vi "Begin.vi"(11 "Image Size":T1=enum."160x120") -> (0 "error out":errorcluster)   [LabVIEW 2012]
doc: "Called before other user functions, this VI is expected to open initial I/O refnums, load in file data, and do all program initialization. Notice that the <B>error out</B> terminal is simply used for data flow. Wiring it to other structures or subVIs ensures that this VI runs first."
uses:
  <vilib>/Rock Robotics/WPI/Camera/WPI_CameraImageSize.ctl
  <vilib>/Rock Robotics/SystemInterfaces/Utilities/FPGA_UtilitiesLED State.ctl
  <vilib>/Rock Robotics/WPI/Joystick/WPI_JoystickDeviceEnum.ctl
  <vilib>/Rock Robotics/SystemInterfaces/DIO/FPGA_DIOChannel.ctl
  <vilib>/Rock Robotics/SystemInterfaces/AI/FPGA_AIChannel.ctl
  <vilib>/Rock Robotics/WPI/Encoder/WPI_EncoderDevRef.ctl
  <vilib>/Rock Robotics/SystemInterfaces/Encoder/FPGA_EncoderIdx.ctl
  <vilib>/Rock Robotics/SystemInterfaces/Counter/FPGA_CounterCtrSystemIndex.ctl
  <vilib>/Rock Robotics/WPI/Encoder/WPI_EncoderType.ctl
  <vilib>/Rock Robotics/WPI/AnalogChannel/WPI_AnalogChannelDevRef.ctl
  <vilib>/Rock Robotics/SystemInterfaces/Typedef/FPGA_TypedefAnalogModule.ctl
  <vilib>/Rock Robotics/WPI/MotorControl/WPI_MotorControlDeviceRef.ctl
  <vilib>/Rock Robotics/SystemInterfaces/Typedef/FPGA_TypedefDigitalModule.ctl
  <vilib>/Rock Robotics/SystemInterfaces/DIO/FPGA_DIOPWMChannel.ctl
  <vilib>/Rock Robotics/WPI/PWM/WPI_PWMDeadband.ctl
  <vilib>/Rock Robotics/WPI/CAN/Jaguar/SubVIs/WPI_CANJaguar_ControlMode.ctl
  <vilib>/Rock Robotics/WPI/PWM/WPI_PWMTransform_ConPane.ctl
  <vilib>/Rock Robotics/SystemInterfaces/Utilities/FPGA_UtilitiesLED Source.ctl
  <vilib>/Utility/file.llb/Read From Spreadsheet File (DBL).vi
  Globals/Pot Home Values.vi
  Globals/Robot Jaguars.vi
  Globals/Encoders Global.vi
  Globals/Potentiometers.vi
  Globals/Are We Calibrating Steering.vi
  Globals/Are We Calibrating Actuator.vi
  Globals/Jaguar Commands.vi
  Globals/Autonomous Joystick Emulation.vi
  Globals/Autonomous Tipping.vi
  Globals/Actuator Home Position.vi
  Globals/Max Tipper Angle.vi
  <vilib>/Rock Robotics/WPI/Camera/WPI_CameraWhite Balance Values.ctl
  <vilib>/Rock Robotics/WPI/Camera/WPI_CameraExposure Values.ctl
  <vilib>/Rock Robotics/WPI/Camera/WPI_CameraFrameRate.ctl
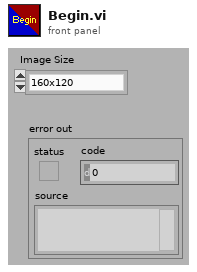
[diagram p1: front panel]
types:
  T1 = typedef "WPI_CameraImageSize.ctl" = enum16{"640x480", "320x240", "160x120"}
  T2 = typedef "FPGA_DIOChannel.ctl" = enum8{"DIO 1", "DIO 2", "DIO 3", "DIO 4", "DIO 5", "DIO 6", "DIO 7", "DIO 8", "DIO 9", "DIO 10", "DIO 11", "DIO 12", "DIO 13", "DIO 14", "Invalid"}
  T3 = typedef "FPGA_TypedefDigitalModule.ctl" = enum16{"Digital Module 1", "Digital Module 2"}
  T4 = typedef "FPGA_AIChannel.ctl" = enum8{"AI 1", "AI 2", "AI 3", "AI 4", "AI 5", "AI 6", "AI 7", "AI 8", "Invalid"}
  T5 = typedef "WPI_EncoderType.ctl" = enum16{"1x", "2x", "4x"}
  T6 = typedef "WPI_MotorControlDeviceRef.ctl" = cluster{"DeviceStatus":errorcluster, "Type":enum16{"PWM", "CAN"}, "PWM":cluster{"Digital Module":T3, "PWM Channel":T7, "DeadBand":T8}, "CAN":cluster{"Device Number":u8, "Control Mode":T9, "Semaphore":T10, "Max Vout":dbl}, "Invert":bool, "TransformRef":T11, "InvTransformRef":T11}
  T7 = typedef "FPGA_DIOPWMChannel.ctl" = enum8{"PWM 1", "PWM 2", "PWM 3", "PWM 4", "PWM 5", "PWM 6", "PWM 7", "PWM 8", "PWM 9", "PWM 10", "Invalid"}
  T8 = typedef "WPI_PWMDeadband.ctl" = cluster{"Name":string, "maxPositivePwm":i32, "minPositivePwm":i32, "centerPwm":i32, "maxNegativePwm":i32, "minNegativePwm":i32, "angularRange":u16}
  T9 = typedef "WPI_CANJaguar_ControlMode.ctl" = enum8{"Percent VBus", "Current", "Speed", "Position", "Voltage"}
  T10 = typedef "Semaphore RefNum" = refnum<k1>
  T11 = typedef "WPI_PWMTransform_ConPane.ctl" = refnum<vi>
  T12 = cluster{"MotorControlDevRef":T6, "MotorControlDevRef":T6, "MotorControlDevRef":T6, "MotorControlDevRef":T6, "MotorControlDevRef":T6, "MotorControlDevRef":T6, "MotorControlDevRef":T6, "MotorControlDevRef":T6}
  T13 = typedef "WPI_AnalogChannelDevRef.ctl" = cluster{"DevStatus":errorcluster, "Analog Module":T14, "Analog Channel":T4}
  T14 = typedef "FPGA_TypedefAnalogModule.ctl" = enum16{"Analog Module 1", "Analog Module 2"}
  T15 = cluster{"Front Left":T13, "Front Right":T13, "Rear Left":T13, "Rear Right":T13, "Actuator":T13}
  T16 = typedef "WPI_EncoderDevRef.ctl" = cluster{"DevStatus":errorcluster, "EncoderIndex":T17, "CounterIndex":T18, "DistancePerCount":dbl, "Decoding Type":T5}
  T17 = typedef "FPGA_EncoderIdx.ctl" = enum8{"Enc 0", "Enc 1", "Enc 2", "Enc 3", "Invalid"}
  T18 = typedef "FPGA_CounterCtrSystemIndex.ctl" = enum8{"Ctr 0", "Ctr 1", "Ctr 2", "Ctr 3", "Ctr 4", "Ctr 5", "Ctr 6", "Ctr 7", "Invalid"}
  T19 = cluster{"Front Left":T16, "Front Right":T16, "Rear Left":T16, "Rear Right":T16, "Shooter":T16}
  T20 = typedef "WPI_JoystickDeviceEnum.ctl" = enum16{"USB 1", "USB 2", "USB 3", "USB 4", "Kinect 1", "Kinect 2"}
  T21 = typedef "FPGA_UtilitiesLED State.ctl" = enum16{"Off", "On", "Toggle"}
  T22 = typedef "FPGA_UtilitiesLED Source.ctl" = enum16{"User LED", "FPGA LED"}
  T23 = typedef "WPI_JoystickDevRef.ctl" = cluster{"Device":T20}
  T24 = typedef "WPI_CameraFrameRate.ctl" = u32
  T25 = typedef "WPI_CameraExposure Values.ctl" = enum16{"Auto", "Flicker-free 50 Hz", "Flicker-free 60 Hz", "Hold current"}
  T26 = typedef "WPI_CameraWhite Balance Values.ctl" = enum16{"Auto", "Fixed indoor", "Fixed outdoor 1", "Fixed outdoor 2", "Fixed fluorescent 1", "Fixed fluorescent 2", "Hold current"}
  T27 = typedef "WPI_CameraDevRef.ctl" = cluster{"Camera Address":string, "CameraStatus":errorcluster, "Acquire Image Notifier":refnum<notifier>}
  T28 = typedef "WPI_DigitalInputDevRef.ctl" = cluster{"DevStatus":errorcluster, "DIO Channel":T2, "Digital Module":T3}
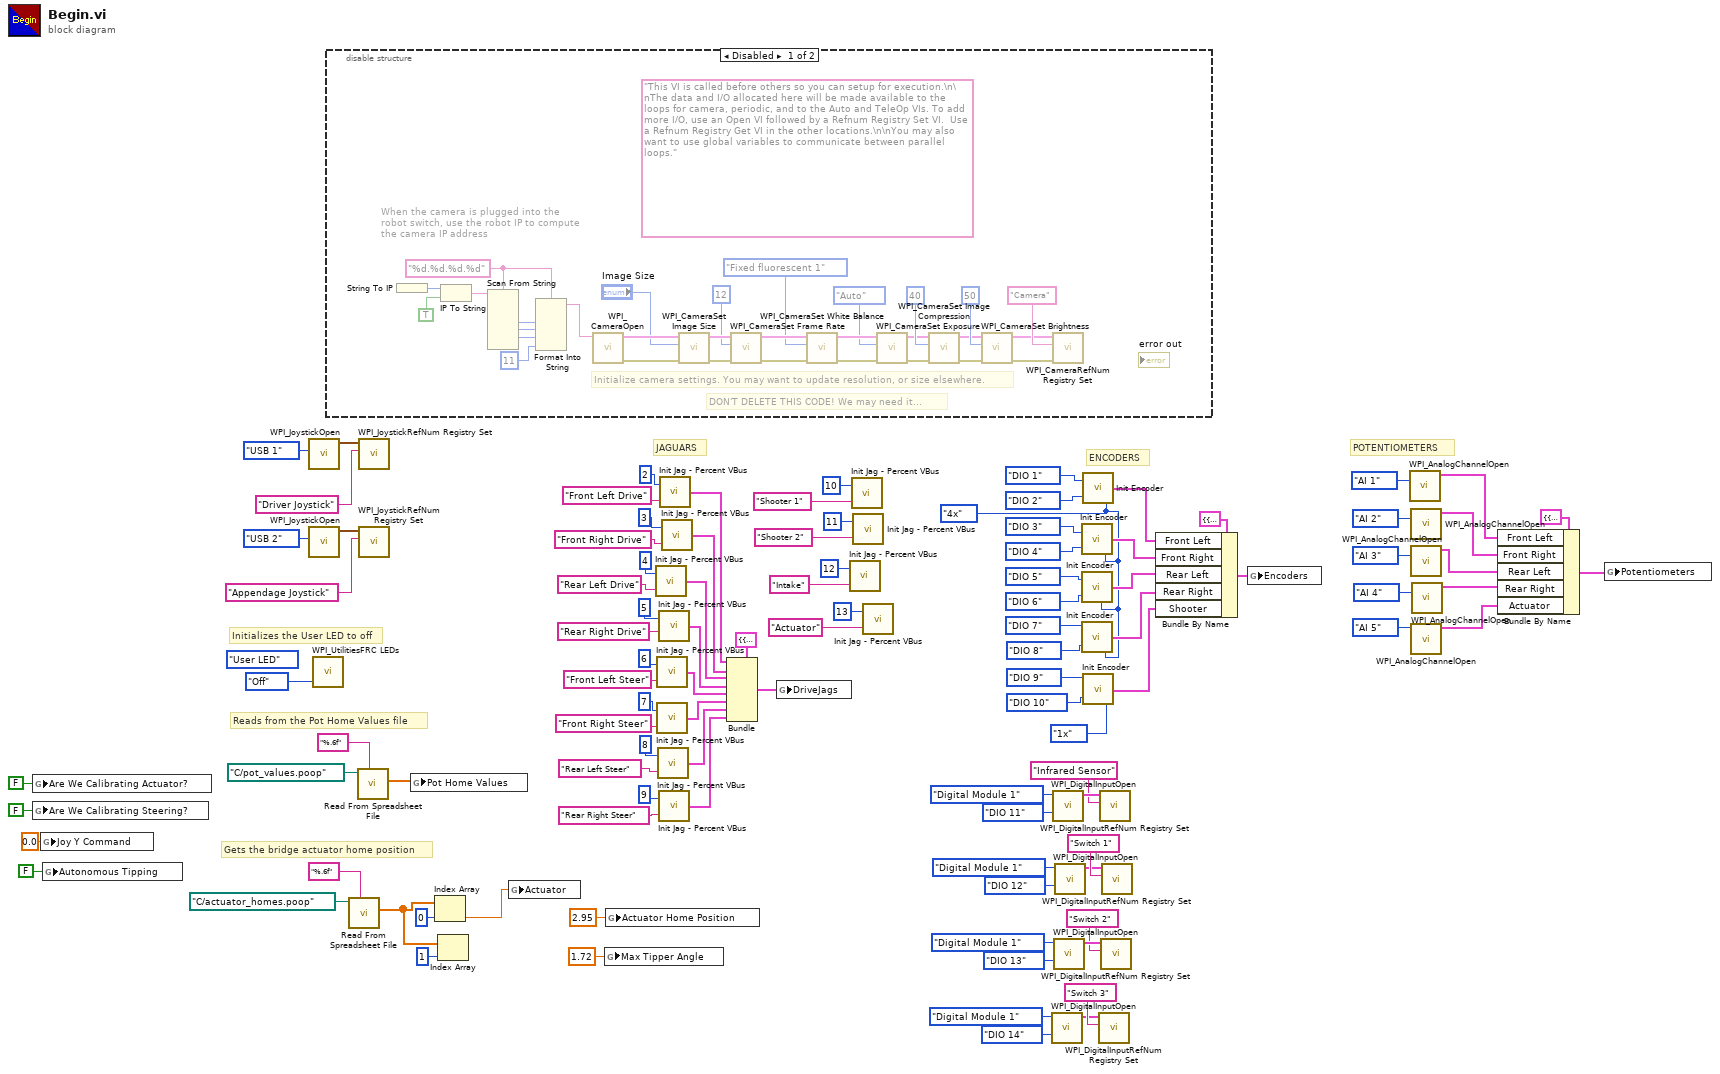
[diagram p0: block diagram]
diagram:
  w64 = WPI_EncoderType."4x" ("Decoding Type")
  (unwired) FPGA_UtilitiesLED_Source."User LED" ("LED Type")
  # "Gets the bridge actuator home position"
  # "JAGUARS"
  # "POTENTIOMETERS"
  # "ENCODERS"
  # "Reads from the Pot Home Values file"
  # "Initializes the User LED to off"
  n1 = global write "Are We Calibrating Actuator.vi" "Are We Calibrating Actuator?"(FALSE ("Are We Calibrating Actuator?")) -> ()
  n2 = global write "Are We Calibrating Steering.vi" "Are We Calibrating Steering?"(FALSE ("Are We Calibrating Steering?")) -> ()
  n3 = global write "Autonomous Joystick Emulation.vi" "Joy Y Command"(0.0 ("Joy Y Command")) -> ()
  n4 = global write "Autonomous Tipping.vi" "Autonomous Tipping"(FALSE ("Autonomous Tipping")) -> ()
  n5 = call <vilib>:"WPI_JoystickOpen.vi"("JoystickDevice"=WPI_JoystickDeviceEnum."USB 1") -> ("JoystickDevRef"=w98:T23)  [unwired: 10 in]
  n6 = call <vilib>:"WPI_JoystickOpen.vi"("JoystickDevice"=WPI_JoystickDeviceEnum."USB 2") -> ("JoystickDevRef"=w95:T23)  [unwired: 10 in]
  n7 = call <vilib>:"WPI_UtilitiesFRC LEDs.vi"("State"=FPGA_UtilitiesLED_State."Off") -> ()  [unwired: 9 in, 2 out]
  n8 = disable-structure shown="Disabled" {
    frame Disabled {
      w105 = "%d.%d.%d.%d" ("format string")
      (unwired) "This VI is called before others so you can setup for execution.\n\nThe data and I/O allocated here will be made available to the loops for camera, periodic, and to the Auto and TeleOp VIs. To add more I/O, use an Open VI followed by a Refnum Registry Set VI.  Use a Refnum Registry Get VI in the other locations.\n\nYou may also want to use global variables to communicate between parallel loops."
      # "DON'T DELETE THIS CODE! We may need it..."
      # "When the camera is plugged into the\nrobot switch, use the robot IP to compute\nthe camera IP address"
      # "Initialize camera settings. You may want to update resolution, or size elsewhere."
      n9 = String To IP() -> (0:w112:u32)  [unwired: 1 in]
      n10 = IP To String(1:TRUE ("dot notation? (F)"), 2:w112) -> (0:w110:string)
      n11 = Scan From String(format string=w105, input string=w110) -> (output 1=w109:i32, output 2=w108:i32, output 3=w107:i32)  [unwired: 7 in, 3 out]
      n12 = Format Into String(format string=w105, w109, w108, w107, 11 ("Compression")) -> (resulting string=w104:string)  [unwired: 2 in, 1 out]
      n13 = call <vilib>:"WPI_CameraOpen.vi"("Camera Address"=w104) -> ("error out"=w124:errorcluster, "CameraDevRef"=w125:T27)  [unwired: 1 in, 8 out]
      n14 = call <vilib>:"WPI_CameraSet Image Size.vi"("error in (no error)"=w124, "Image Size"="Image Size", "CameraDevRef"=w125) -> ("error out"=w123:errorcluster, "CameraDevRef Out"=w126:T27)  [unwired: 7 out]
      n15 = call <vilib>:"WPI_CameraSet Frame Rate.vi"("error in (no error)"=w123, "Frame Rate (fps)"=T24 12, "CameraDevRef"=w126) -> ("error out"=w122:errorcluster, "CameraDevRef Out"=w128:T27)  [unwired: 7 out]
      n16 = call <vilib>:"WPI_CameraSet White Balance.vi"("error in (no error)"=w122, "White Balance"=WPI_CameraWhite_Balance_Values."Fixed fluorescent 1", "CameraDevRef"=w128) -> ("error out"=w121:errorcluster, "CameraDevRef Out"=w127:T27)  [unwired: 7 out]
      n17 = call <vilib>:"WPI_CameraSet Exposure.vi"("error in (no error)"=w121, "Exposure"=WPI_CameraExposure_Values."Auto", "CameraDevRef"=w127) -> ("error out"=w120:errorcluster, "CameraDevRef Out"=w130:T27)  [unwired: 7 out]
      n18 = call <vilib>:"WPI_CameraSet Image Compression.vi"("error in (no error)"=w120, "Compression"=40, "CameraDevRef"=w130) -> ("error out"=w119:errorcluster, "CameraDevRef Out"=w129:T27)  [unwired: 7 out]
      n19 = call <vilib>:"WPI_CameraSet Brightness.vi"("error in (no error)"=w119, "Brightness"=50, "CameraDevRef"=w129) -> ("error out"=w117:errorcluster, "CameraDevRef Out"=w118:T27)  [unwired: 7 out]
      n20 = call <vilib>:"WPI_CameraRefNum Registry Set.vi"("error in (no error)"=w117, "refnum name"="Camera", "CameraDevRef"=w118) -> ()  [unwired: 9 out]
    }
    frame Enabled {
    }
  }
  n21 = call-poly <vilib>:"Read From Spreadsheet File.vi"("format (%.3f)"="%.6f", "file path (dialog if empty)"=path "C:/actuator_homes.poop") -> ("first row"=w35:dbl[])  [unwired: 5 in, 4 out]
  n22 = call-poly <vilib>:"Read From Spreadsheet File.vi"("format (%.3f)"="%.6f", "file path (dialog if empty)"=path "C:/pot_values.poop") -> ("first row"=w100:dbl[])  [unwired: 5 in, 4 out]
  n23 = call <vilib>:"WPI_JoystickRefNum Registry Set.vi"("refnum name"="Driver Joystick", "JoystickDevRef"=w98) -> ()  [unwired: 8 in, 2 out]
  n24 = call <vilib>:"WPI_JoystickRefNum Registry Set.vi"("refnum name"="Appendage Joystick", "JoystickDevRef"=w95) -> ()  [unwired: 8 in, 2 out]
  n25 = global write "Pot Home Values.vi" "Pot Home Values"(w100) -> ()
  n26 = Index Array(array=w35, index=0) -> (element=w33:dbl)
  n27 = Index Array(array=w35, index=1) -> ()  [unwired: 1 out]
  n28 = global write "Jaguar Commands.vi" "Actuator"(w33) -> ()
  n29 = global write "Max Tipper Angle.vi" "Max Tipper Angle"(1.72 ("Max Tipper Angle")) -> ()
  n30 = global write "Actuator Home Position.vi" "Actuator Home Position"(2.95 ("Actuator Home Position")) -> ()
  n31 = call "Init Jag - Percent VBus.vi"("Jag Refnum Name"="Rear Left Drive", "Device Number"=u8 4) -> ("MotorControlDevRef"=w54:T6)
  n32 = call "Init Jag - Percent VBus.vi"("Jag Refnum Name"="Front Left Steer", "Device Number"=u8 6) -> ("MotorControlDevRef"=w3:T6)
  n33 = call "Init Jag - Percent VBus.vi"("Jag Refnum Name"="Front Right Steer", "Device Number"=u8 7) -> ("MotorControlDevRef"=w4:T6)
  n34 = call "Init Jag - Percent VBus.vi"("Jag Refnum Name"="Rear Left Steer", "Device Number"=u8 8) -> ("MotorControlDevRef"=w6:T6)
  n35 = call "Init Jag - Percent VBus.vi"("Jag Refnum Name"="Rear Right Drive", "Device Number"=u8 5) -> ("MotorControlDevRef"=w51:T6)
  n36 = call "Init Jag - Percent VBus.vi"("Jag Refnum Name"="Rear Right Steer", "Device Number"=u8 9) -> ("MotorControlDevRef"=w5:T6)
  n37 = call "Init Jag - Percent VBus.vi"("Jag Refnum Name"="Front Left Drive", "Device Number"=u8 2) -> ("MotorControlDevRef"=w62:T6)
  n38 = call "Init Jag - Percent VBus.vi"("Jag Refnum Name"="Front Right Drive", "Device Number"=u8 3) -> ("MotorControlDevRef"=w57:T6)
  n39 = Bundle(cluster=T12 {"MotorControlDevRef"={"DeviceStatus"={"status"=FALSE, "code"=0, "source"=""}, "Type"=enum."PWM", "PWM"={"Digital Module"=enum."Digital Module 1", "PWM Channel"=enum."PWM 1", "DeadBand"={"Name"="", "maxPositivePwm"=0, "minPositivePwm"=0, "centerPwm"=0, "maxNegativePwm"=0, "minNegativePwm"=0, "angularRange"=0}}, "CAN"={"Device Number"=0, "Control Mode"=enum."Percent VBus", "Semaphore"=refnum, "Max Vout"=0.0}, "Invert"=FALSE, "TransformRef"=refnum, "InvTransformRef"=refnum}, "MotorControlDevRef"={"DeviceStatus"={"status"=FALSE, "code"=0, "source"=""}, "Type"=enum."PWM", "PWM"={"Digital Module"=enum."Digital Module 1", "PWM Channel"=enum."PWM 1", "DeadBand"={"Name"="", "maxPositivePwm"=0, "minPositivePwm"=0, "centerPwm"=0, "maxNegativePwm"=0, "minNegativePwm"=0, "angularRange"=0}}, "CAN"={"Device Number"=0, "Control Mode"=enum."Percent VBus", "Semaphore"=refnum, "Max Vout"=0.0}, "Invert"=FALSE, "TransformRef"=refnum, "InvTransformRef"=refnum}, "MotorControlDevRef"={"DeviceStatus"={"status"=FALSE, "code"=0, "source"=""}, "Type"=enum."PWM", "PWM"={"Digital Module"=enum."Digital Module 1", "PWM Channel"=enum."PWM 1", "DeadBand"={"Name"="", "maxPositivePwm"=0, "minPositivePwm"=0, "centerPwm"=0, "maxNegativePwm"=0, "minNegativePwm"=0, "angularRange"=0}}, "CAN"={"Device Number"=0, "Control Mode"=enum."Percent VBus", "Semaphore"=refnum, "Max Vout"=0.0}, "Invert"=FALSE, "TransformRef"=refnum, "InvTransformRef"=refnum}, "MotorControlDevRef"={"DeviceStatus"={"status"=FALSE, "code"=0, "source"=""}, "Type"=enum."PWM", "PWM"={"Digital Module"=enum."Digital Module 1", "PWM Channel"=enum."PWM 1", "DeadBand"={"Name"="", "maxPositivePwm"=0, "minPositivePwm"=0, "centerPwm"=0, "maxNegativePwm"=0, "minNegativePwm"=0, "angularRange"=0}}, "CAN"={"Device Number"=0, "Control Mode"=enum."Percent VBus", "Semaphore"=refnum, "Max Vout"=0.0}, "Invert"=FALSE, "TransformRef"=refnum, "InvTransformRef"=refnum}, "MotorControlDevRef"={"DeviceStatus"={"status"=FALSE, "code"=0, "source"=""}, "Type"=enum."PWM", "PWM"={"Digital Module"=enum."Digital Module 1", "PWM Channel"=enum."PWM 1", "DeadBand"={"Name"="", "maxPositivePwm"=0, "minPositivePwm"=0, "centerPwm"=0, "maxNegativePwm"=0, "minNegativePwm"=0, "angularRange"=0}}, "CAN"={"Device Number"=0, "Control Mode"=enum."Percent VBus", "Semaphore"=refnum, "Max Vout"=0.0}, "Invert"=FALSE, "TransformRef"=refnum, "InvTransformRef"=refnum}, "MotorControlDevRef"={"DeviceStatus"={"status"=FALSE, "code"=0, "source"=""}, "Type"=enum."PWM", "PWM"={"Digital Module"=enum."Digital Module 1", "PWM Channel"=enum."PWM 1", "DeadBand"={"Name"="", "maxPositivePwm"=0, "minPositivePwm"=0, "centerPwm"=0, "maxNegativePwm"=0, "minNegativePwm"=0, "angularRange"=0}}, "CAN"={"Device Number"=0, "Control Mode"=enum."Percent VBus", "Semaphore"=refnum, "Max Vout"=0.0}, "Invert"=FALSE, "TransformRef"=refnum, "InvTransformRef"=refnum}, "MotorControlDevRef"={"DeviceStatus"={"status"=FALSE, "code"=0, "source"=""}, "Type"=enum."PWM", "PWM"={"Digital Module"=enum."Digital Module 1", "PWM Channel"=enum."PWM 1", "DeadBand"={"Name"="", "maxPositivePwm"=0, "minPositivePwm"=0, "centerPwm"=0, "maxNegativePwm"=0, "minNegativePwm"=0, "angularRange"=0}}, "CAN"={"Device Number"=0, "Control Mode"=enum."Percent VBus", "Semaphore"=refnum, "Max Vout"=0.0}, "Invert"=FALSE, "TransformRef"=refnum, "InvTransformRef"=refnum}, "MotorControlDevRef"={"DeviceStatus"={"status"=FALSE, "code"=0, "source"=""}, "Type"=enum."PWM", "PWM"={"Digital Module"=enum."Digital Module 1", "PWM Channel"=enum."PWM 1", "DeadBand"={"Name"="", "maxPositivePwm"=0, "minPositivePwm"=0, "centerPwm"=0, "maxNegativePwm"=0, "minNegativePwm"=0, "angularRange"=0}}, "CAN"={"Device Number"=0, "Control Mode"=enum."Percent VBus", "Semaphore"=refnum, "Max Vout"=0.0}, "Invert"=FALSE, "TransformRef"=refnum, "InvTransformRef"=refnum}}, "MotorControlDevRef"=w62, "MotorControlDevRef"=w57, "MotorControlDevRef"=w54, "MotorControlDevRef"=w51, "MotorControlDevRef"=w3, "MotorControlDevRef"=w4, "MotorControlDevRef"=w6, "MotorControlDevRef"=w5) -> (w68:T12)
  n40 = global write "Robot Jaguars.vi" "DriveJags"(w68) -> ()
  n41 = call "Init Jag - Percent VBus.vi"("Jag Refnum Name"="Intake" ("refnum name"), "Device Number"=u8 12) -> ()  [unwired: 1 out]
  n42 = call "Init Jag - Percent VBus.vi"("Jag Refnum Name"="Shooter 1" ("refnum name"), "Device Number"=u8 10) -> ()  [unwired: 1 out]
  n43 = call "Init Jag - Percent VBus.vi"("Jag Refnum Name"="Shooter 2" ("refnum name"), "Device Number"=u8 11) -> ()  [unwired: 1 out]
  n44 = call "Init Jag - Percent VBus.vi"("Jag Refnum Name"="Actuator" ("refnum name"), "Device Number"=u8 13) -> ()  [unwired: 1 out]
  n45 = call <vilib>:"WPI_DigitalInputOpen.vi"("DIO Channel"=FPGA_DIOChannel."DIO 14", "Digital Module (Module 1)"=FPGA_TypedefDigitalModule."Digital Module 1") -> ("DigitalInputDevRef"=w15:T28)  [unwired: 8 in, 1 out]
  n46 = call <vilib>:"WPI_DigitalInputOpen.vi"("DIO Channel"=FPGA_DIOChannel."DIO 11", "Digital Module (Module 1)"=FPGA_TypedefDigitalModule."Digital Module 1") -> ("DigitalInputDevRef"=w32:T28)  [unwired: 8 in, 1 out]
  n47 = call <vilib>:"WPI_DigitalInputOpen.vi"("DIO Channel"=FPGA_DIOChannel."DIO 13", "Digital Module (Module 1)"=FPGA_TypedefDigitalModule."Digital Module 1") -> ("DigitalInputDevRef"=w22:T28)  [unwired: 8 in, 1 out]
  n48 = call <vilib>:"WPI_DigitalInputOpen.vi"("DIO Channel"=FPGA_DIOChannel."DIO 12", "Digital Module (Module 1)"=FPGA_TypedefDigitalModule."Digital Module 1") -> ("DigitalInputDevRef"=w23:T28)  [unwired: 8 in, 1 out]
  n49 = call "Init Encoder.vi"("DIO Channel A"=FPGA_DIOChannel."DIO 3", "DIO Channel B"=FPGA_DIOChannel."DIO 4", "Decoding Type"=w64) -> ("EncoderDevRef"=w75:T16)  [unwired: 1 in]
  n50 = call "Init Encoder.vi"("DIO Channel A"=FPGA_DIOChannel."DIO 5", "DIO Channel B"=FPGA_DIOChannel."DIO 6", "Decoding Type"=w64) -> ("EncoderDevRef"=w74:T16)  [unwired: 1 in]
  n51 = call "Init Encoder.vi"("DIO Channel A"=FPGA_DIOChannel."DIO 7", "DIO Channel B"=FPGA_DIOChannel."DIO 8", "Decoding Type"=w64) -> ("EncoderDevRef"=w73:T16)  [unwired: 1 in]
  n52 = call "Init Encoder.vi"("DIO Channel A"=FPGA_DIOChannel."DIO 1", "DIO Channel B"=FPGA_DIOChannel."DIO 2", "Decoding Type"=w64) -> ("EncoderDevRef"=w76:T16)  [unwired: 1 in]
  n53 = call "Init Encoder.vi"("DIO Channel A"=FPGA_DIOChannel."DIO 9", "DIO Channel B"=FPGA_DIOChannel."DIO 10", "Decoding Type"=WPI_EncoderType."1x") -> ("EncoderDevRef"=w65:T16)  [unwired: 1 in]
  n54 = call <vilib>:"WPI_DigitalInputRefNum Registry Set.vi"("refnum name"="Switch 3", "DigitalInputDevRef"=w15) -> ()  [unwired: 8 in, 2 out]
  n55 = call <vilib>:"WPI_DigitalInputRefNum Registry Set.vi"("refnum name"="Infrared Sensor", "DigitalInputDevRef"=w32) -> ()  [unwired: 8 in, 2 out]
  n56 = call <vilib>:"WPI_DigitalInputRefNum Registry Set.vi"("refnum name"="Switch 2", "DigitalInputDevRef"=w22) -> ()  [unwired: 8 in, 2 out]
  n57 = call <vilib>:"WPI_DigitalInputRefNum Registry Set.vi"("refnum name"="Switch 1", "DigitalInputDevRef"=w23) -> ()  [unwired: 8 in, 2 out]
  n58 = Bundle By Name(cluster=T19 {"Front Left"={"DevStatus"={"status"=FALSE, "code"=0, "source"=""}, "EncoderIndex"=enum."Invalid", "CounterIndex"=enum."Invalid", "DistancePerCount"=1.0, "Decoding Type"=enum."4x"}, "Front Right"={"DevStatus"={"status"=FALSE, "code"=0, "source"=""}, "EncoderIndex"=enum."Invalid", "CounterIndex"=enum."Invalid", "DistancePerCount"=1.0, "Decoding Type"=enum."4x"}, "Rear Left"={"DevStatus"={"status"=FALSE, "code"=0, "source"=""}, "EncoderIndex"=enum."Invalid", "CounterIndex"=enum."Invalid", "DistancePerCount"=1.0, "Decoding Type"=enum."4x"}, "Rear Right"={"DevStatus"={"status"=FALSE, "code"=0, "source"=""}, "EncoderIndex"=enum."Invalid", "CounterIndex"=enum."Invalid", "DistancePerCount"=1.0, "Decoding Type"=enum."4x"}, "Shooter"={"DevStatus"={"status"=FALSE, "code"=0, "source"=""}, "EncoderIndex"=enum."Invalid", "CounterIndex"=enum."Invalid", "DistancePerCount"=1.0, "Decoding Type"=enum."4x"}} ("Encoders"), "Front Left"=w76, "Front Right"=w75, "Rear Left"=w74, "Rear Right"=w73, "Shooter"=w65) -> (w71:T19)
  n59 = global write "Encoders Global.vi" "Encoders"(w71) -> ()
  n60 = call <vilib>:"WPI_AnalogChannelOpen.vi"("Analog Channel"=FPGA_AIChannel."AI 1") -> ("AIDeviceRef"=w91:T13)  [unwired: 9 in, 1 out]
  n61 = call <vilib>:"WPI_AnalogChannelOpen.vi"("Analog Channel"=FPGA_AIChannel."AI 2") -> ("AIDeviceRef"=w87:T13)  [unwired: 9 in, 1 out]
  n62 = call <vilib>:"WPI_AnalogChannelOpen.vi"("Analog Channel"=FPGA_AIChannel."AI 3") -> ("AIDeviceRef"=w86:T13)  [unwired: 9 in, 1 out]
  n63 = call <vilib>:"WPI_AnalogChannelOpen.vi"("Analog Channel"=FPGA_AIChannel."AI 5") -> ("AIDeviceRef"=w45:T13)  [unwired: 9 in, 1 out]
  n64 = call <vilib>:"WPI_AnalogChannelOpen.vi"("Analog Channel"=FPGA_AIChannel."AI 4") -> ("AIDeviceRef"=w85:T13)  [unwired: 9 in, 1 out]
  n65 = Bundle By Name(cluster=T15 {"Front Left"={"DevStatus"={"status"=FALSE, "code"=0, "source"=""}, "Analog Module"=enum."Analog Module 1", "Analog Channel"=enum."Invalid"}, "Front Right"={"DevStatus"={"status"=FALSE, "code"=0, "source"=""}, "Analog Module"=enum."Analog Module 1", "Analog Channel"=enum."Invalid"}, "Rear Left"={"DevStatus"={"status"=FALSE, "code"=0, "source"=""}, "Analog Module"=enum."Analog Module 1", "Analog Channel"=enum."Invalid"}, "Rear Right"={"DevStatus"={"status"=FALSE, "code"=0, "source"=""}, "Analog Module"=enum."Analog Module 1", "Analog Channel"=enum."Invalid"}, "Actuator"={"DevStatus"={"status"=FALSE, "code"=0, "source"=""}, "Analog Module"=enum."Analog Module 1", "Analog Channel"=enum."Invalid"}} ("Potentiometers"), "Front Left"=w91, "Front Right"=w87, "Rear Left"=w86, "Rear Right"=w85, "Actuator"=w45) -> (w92:T15)
  n66 = global write "Potentiometers.vi" "Potentiometers"(w92) -> ()
